vi "SiosIfmSetBlockMode.vi"(1 "Measurement Flags":i32(ring) items=["IFM_MEAS_TWOCHANNEL"=758, "IFM_MEAS_THREECHANNEL"=1792, "IFM_MEAS_FOURCHANNEL"=3840, "IFM_MEAS_CH1 | IFM_MEAS_ONECHANNEL"=256, "IFM_MEAS_CH2"=512, "IFM_MEAS_CH3"=1024, "IFM_MEAS_CH4"=2048, "IFM_MEAS_USERMODE"=1, "IFM_MEAS_LENGTH"=2, "IFM_MEAS_SINCOS"=4, "IFM_MEAS_CIRCLE"=8, "IFM_MEAS_PATTERN"=16, "IFM_MEAS_CLOCKCOUNT | IFM_MEAS_VAL_COUNTER"=32, "IFM_MEAS_SAMPLECOUNT"=128, "IFM_MEAS_VAL_MASK"=63, "IFM_MEAS_BEAMBREAK_OFF"=64, "IFM_MEAS_FILTER_DEFAULT"=0, "IFM_MEAS_FILTER_OFF"=4096, "IFM_MEAS_FILTER_USER"=8192, "IFM_MEAS_FILTER_MASK"=12288, "IFM_MEAS_RAWMODE"=16384], 2 "Trigger Mode":i32(ring) items=["IFM_TRIGGER_OFF"=0, "IFM_TRIGGER_START"=1, "IFM_TRIGGER_STARTSTOP_PROC"=2, "IFM_TRIGGER_STARTSTOP"=4, "IFM_TRIGGER_CLOCK"=8, "IFM_TRIGGER_EVENT"=10, "IFM_TRIGGER_CLOCK_RISING_EDGE"=256, "IFM_TRIGGER_STARTSTOP_RISING_EDGE"=512, "IFM_TRIGGER_EVENT_RISING_EDGE"=1024], 3 "Output Wordrate":i32, 4 "Device Number":i32) -> (0 "Success":i32)   [LabVIEW 2009]
uses:
  siosifm.dll
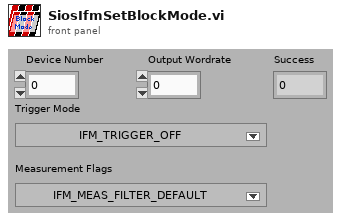
[diagram p1: front panel]
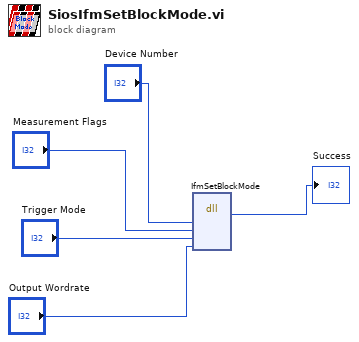
[diagram p0: block diagram]
diagram:
  n1 = dll-call lib="C:/WORK/Artem/RE-10/SIOS_IfmDLL/siosifm.dll" fn="IfmSetBlockMode"("devNumber"="Device Number", "measurementFlags"="Measurement Flags", "triggerMode"="Trigger Mode", "outputWordRate"="Output Wordrate") -> ("Success"=→"Success":i32)  [unwired: 7 in, 2 out]
